vi "Set_2400_to_Autorange.vi"() -> ()   [LabVIEW 2020]
uses:
  <instrlib>/Keithley 24XX/Keithley 24XX.lvlib
panel:
  in  "Function (0: Volts)":u16(ring) items=["Volts", "Current", "Resistance"]
  out "error out":errorcluster
  in  "error in (no error)":errorcluster
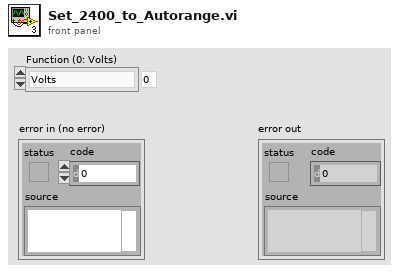
[diagram p1: front panel]
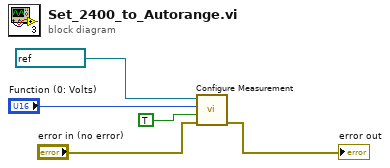
[diagram p0: block diagram]
diagram:
  n1 = call <instrlib>:"Configure Measurement.vi"("error in (no error)"="error in (no error)", "Enable Auto Range (T:Enable)"=TRUE, "Function (0: Volts)"="Function (0: Volts)", "VISA resource name"=refnum<visa-resource-name> "Keithley") -> ("error out"=→"error out":errorcluster)  [unwired: 6 in, 1 out]
